vi "Read FGV DataOut.vi"(7 "TSt/FConveyor":bool, 8 "error in (no error)":errorcluster, 10 "Data":T1, 11 "LineScan in":refnum<class "LineScan.lvclass">) -> (0 "error out":errorcluster, 2 "DataOut":string, 3 "LineScan out":refnum<class "LineScan.lvclass">)   [LabVIEW 2019, in "LineScan.lvclass"]
uses:
  LineScan.lvclass
  Ctrl/Auto Inspection Data Name.ctl
  Ctrl/Auto Inspection Station Name2.ctl
panel:
  out "Numeric":i32
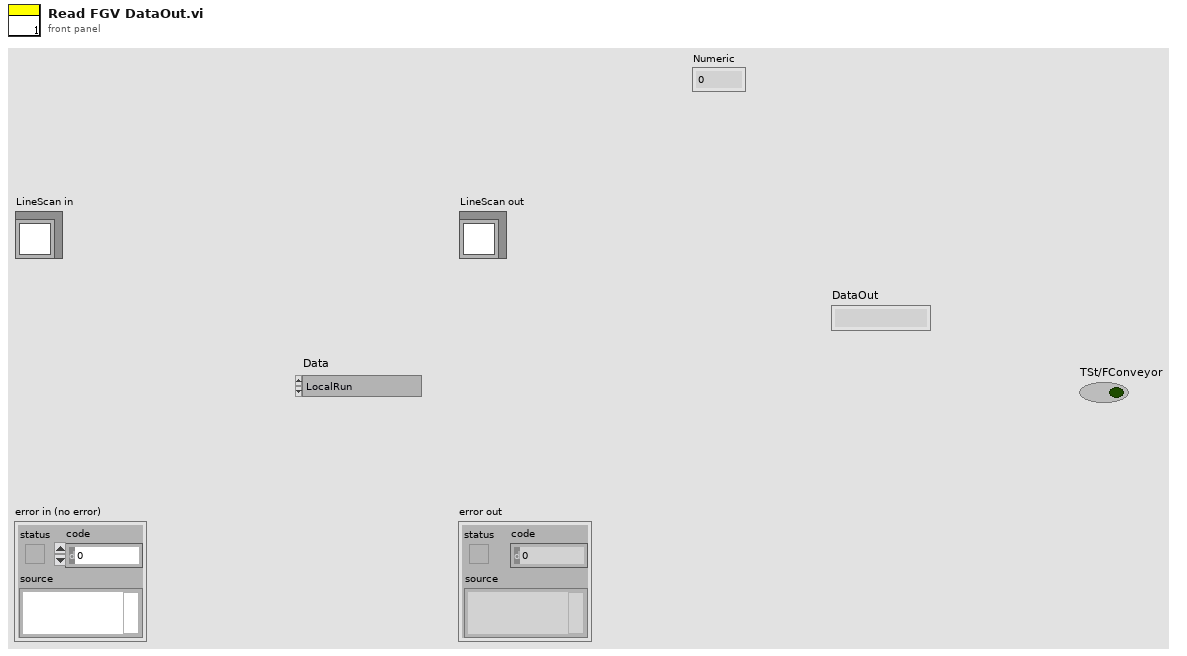
[diagram p1: front panel]
types:
  T1 = typedef "Auto Inspection Data Name.ctl" = enum16{"LocalRun", "ItemSN(TimeCode)", "CurrentAction", "Error", "Data", "OKNG", "電壓值", "電壓值判斷", "電流值", "電流值判斷", "Laser1 Data", "Laser2 Data", "Laser OKNG", "StationNO"}
  T2 = typedef "Auto Inspection Station Name2.ctl" = enum16{"S1Barcode", "S2Measure", "S3Measure", "S4Measure", "S5Measure", "S11_LaserCheck", "S8_Vision AI"}
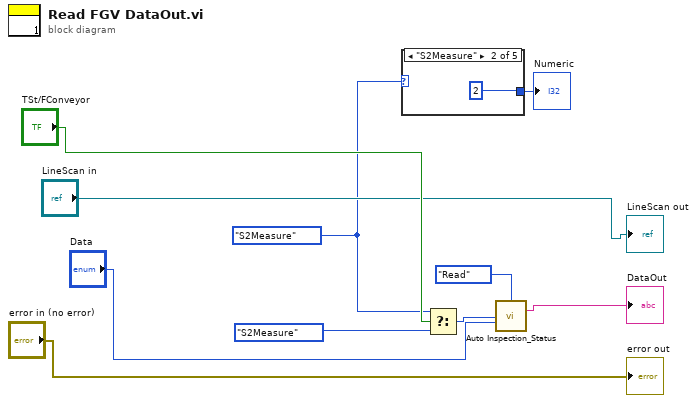
[diagram p0: block diagram]
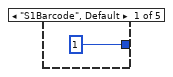
[diagram p2: hidden frame]
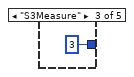
[diagram p3: hidden frame]
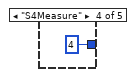
[diagram p4: hidden frame]
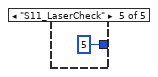
[diagram p5: hidden frame]
diagram:
  w2 = Auto_Inspection_Station_Name2."S2Measure" ("Station")
  n1 = case shown="\"S2Measure\"" w2 {
    tunnel: [1 2 3 4 5] -> w1
    frame "S1Barcode", Default {
    }
    frame "S2Measure" {
    }
    frame "S3Measure" {
    }
    frame "S4Measure" {
    }
    frame "S11_LaserCheck" {
    }
  }
  "Numeric" <- w1
  n2 = Select(t=w2, s="TSt/FConveyor", f=Auto_Inspection_Station_Name2."S2Measure" ("Station")) -> (s? t:f=w8:T2)
  n3 = call "Auto Inspection_Status.vi"("Action"=enum16{"Initial", "Write", "Read"}."Read", "Station"=w8, "Data"="Data") -> ("DataOut"=→"DataOut":string)  [unwired: 10 in, 2 out]
  "error out" <- "error in (no error)"
  "LineScan out" <- "LineScan in"
